vi "Vision Research Phantom Series PhCon PhNVMSetSaveRange.vi"(0 "CN in":u32=1, 2 "pRng":T1, 5 "Error In (no error)":errorcluster) -> (14 "CN out":u32=1, 19 "Error Out":errorcluster)   [LabVIEW 2013, in "VRI.lvlib"]
doc: "PhCon.dll\n\nPhNVMSetSaveRange\nHRESULT PhNVMSetSaveRange(UINT CN, PIMRANGE pRng);\n\nParameters Description\nCN (in) Camera number\npRng (in) Image range\nReturn HRESULT (0=Ok)\nComments Sets the save range for the NVM Save using \n PHNVMSave or NVM continuous recording. It does\n not change the range saved by PhNVMSaveClip."
uses:
  VRI.lvlib
  _Type Defs/PHCon IMRANGE.ctl
  Phantom DLLs/PhCon.dll
panel:
  # "For instructions on the use of this VI, press Ctrl+H to display the help window and move the mouse over the icon, controls, and indicators"
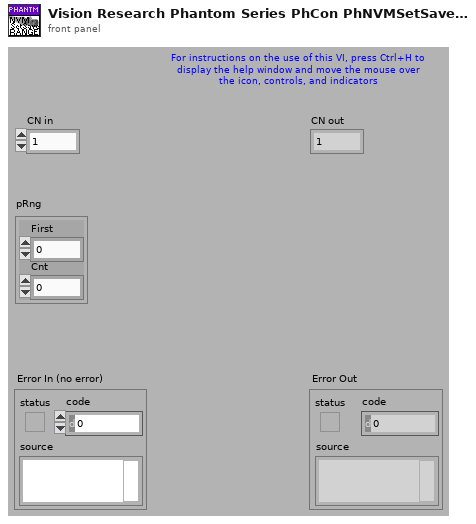
[diagram p1: front panel]
types:
  T1 = typedef "VRI.lvlib/PHCon IMRANGE.ctl" = cluster{"First":i32, "Cnt":u32}
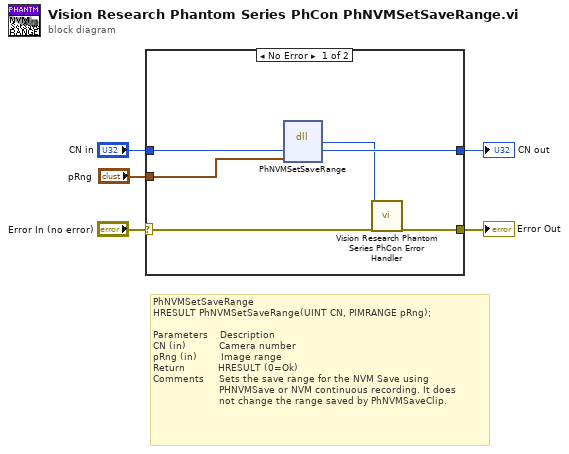
[diagram p0: block diagram]
diagram:
  # "PhNVMSetSaveRange\nHRESULT PhNVMSetSaveRange(UINT CN, PIMRANGE pRng);\n\nParameters    Description\nCN (in)           Camera number\npRng (in)        Image range\nReturn           HRESULT (0=Ok)\nComments     Sets the save range for the NVM Save using \n                      PHNVMSave or NVM continuous recording. It does\n                      not change the range saved by PhNVMSaveClip."
  n1 = case shown="No Error" "Error In (no error)" {
    selector: "Error In (no error)" -> [w11 w13]
    tunnel: [w10 w13] -> w4
    tunnel: "CN in" -> [w9 w12]
    tunnel: [w8 w12] -> w2
    tunnel: "pRng" -> [w7 _]
    frame No Error {
      n2 = dll-call lib="C:/Projects/SDK/32-bit/Vision Research Phantom Series Labview Driver/Phantom DLLs/PhCon.dll" fn="PhNVMSetSaveRange"("CN"=w9, "pRng"=w7) -> ("HRESULT"=w6:i32, "CN"=w8:u32)  [unwired: 4 in, 2 out]
      n3 = call "Vision Research Phantom Series PhCon Error Handler.vi"("ErrNo"=w6, "Error In (no error)"=w11) -> ("Error Out"=w10:errorcluster)  [unwired: 17 out]
    }
    frame Error {
    }
  }
  "Error Out" <- w4
  "CN out" <- w2
